vi "Actor Core.vi"(8 "error in":errorcluster, 11 "[V]Waveform Display in":refnum<class "[V]Waveform Display.lvclass">) -> (0 "error out":errorcluster, 3 "Actor out":refnum<class "Actor.lvclass">)   [LabVIEW 2020, in "[V]Waveform Display.lvlib" / "[V]Waveform Display.lvclass"]
doc: "(<B>Filename</B>: Actor Framework.lvlib:Actor.lvclass:Actor Core.vi)\n\nReceives messages to the actor, reacts to them, and initiates any error handling that may shut the actor down.\n\nDescendant classes may override this VI to append parallel tasks for the actor to complete while it handles messages. Overrides use the Call Parent Class Method node."
uses:
  [V]Waveform Display.lvclass
  <vilib>/ActorFramework/Actor/Actor.lvclass
  Depden On/Abstruct View/Abstruct View/Abstruct View.lvclass/Abstruct View.ctl
  [V]Waveform Display.lvclass/[V]Waveform Display.ctl
  Depden On/Abstruct View/Abstruct View/Data Accessors/Write Core VI.vi
  Depden On/MVVM Framework/MVVM Abstruct View/MVVM Abstruct View/MVVM Abstruct View.lvclass
panel:
  out "System Waveform Chart":waveform(dbl)[](graph)
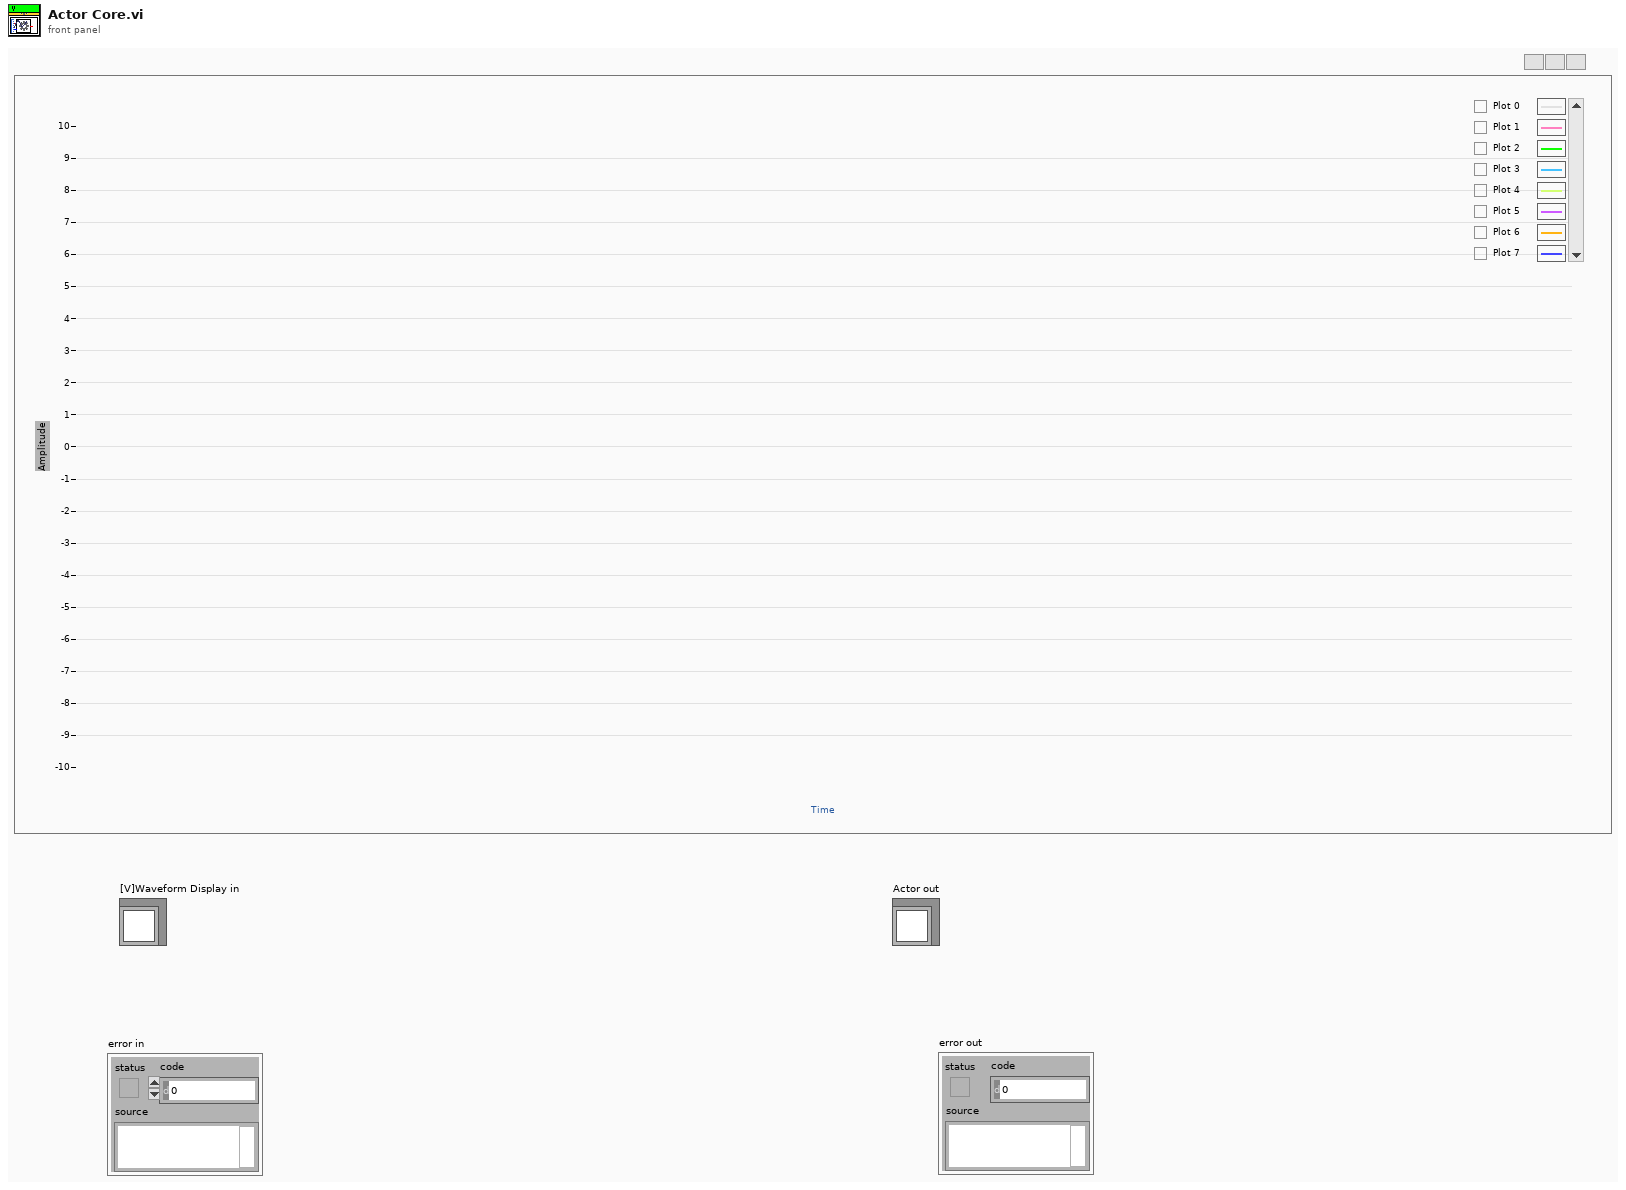
[diagram p1: front panel]
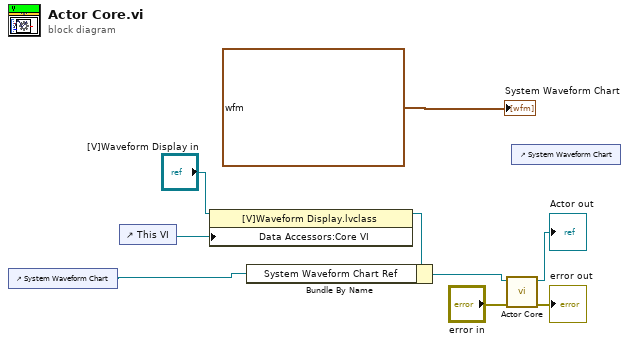
[diagram p0: block diagram]
diagram:
  n1 = control-ref of="System Waveform Chart"() -> (w2:refnum<vi>)
  n2 = control-ref of="This VI"() -> (w3:refnum<vi>)
  n3 = property class="[V]Waveform Display.lvclass"(reference="[V]Waveform Display in", "Data Accessors:Core VI"=w3) -> (reference out=w4:refnum<class "[V]Waveform Display.lvclass">)  [unwired: 1 in, 1 out]
  n4 = Bundle By Name(cluster=w4, "System Waveform Chart Ref"=w2) -> (w6:refnum<class "[V]Waveform Display.lvclass">)
  n5 = call-parent "Actor Core.vi"("error in"="error in", "Abstruct View in"=w6) -> ("error out"=→"error out":errorcluster, "Actor out"=→"Actor out":refnum<class "Actor.lvclass">)  [unwired: 8 in]
  n6 = control-ref of="System Waveform Chart"() -> ()  [unwired: 1 out]
  "System Waveform Chart" <- waveform(dbl)[] [{"t0"=timestamp(0 s since 1904-01-01), "dt"=1.0, "Y"=[0.0]}] ("System Waveform Chart")
